vi "Create.vi"(6 "Shared Library":path=path "", 7 "Flags":i32, 8 "Error In":errorcluster) -> (0 "Error Out":errorcluster, 3 "LabSSH2":refnum<class "Context.lvclass">)   [LabVIEW 2017, in "LabSSH2.lvlib" / "Context.lvclass"]
uses:
  Context.lvclass
  Context.lvclass/Context.ctl
  LabSSH2.lvlib
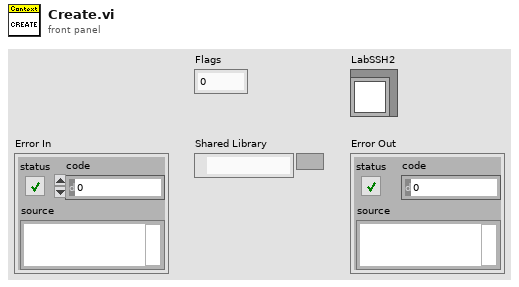
[diagram p1: front panel]
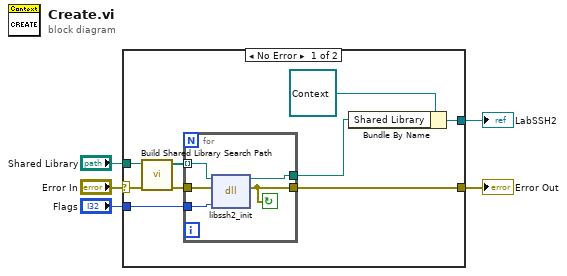
[diagram p0: block diagram]
diagram:
  n1 = case shown="No Error" "Error In" {
    selector: "Error In" -> [w14 w20]
    tunnel: "Shared Library" -> [w13 _]
    tunnel: [w7 w20] -> w3
    tunnel: [w8 _] -> w2
    tunnel: "Flags" -> [w6 _]
    frame No Error {
      n2 = call "Build Shared Library Search Path.vi"("Error In"=w14, "libssh2 Shared Library"=w13) -> ("Error Out"=w11:errorcluster, "Search Path"=w12:path[])  [unwired: 8 in]
      n3 = for {
        tunnel: w12 -> [w18] mode=indexing
        tunnel: w11 -> [w19]
        tunnel: [w17] -> w9
        tunnel: [w16] -> w7
        tunnel: w6 -> [w15]
        stop <- w16 continue-if-true
        n4 = dll-call lib="C:/Program Files/libssh2/bin/libssh2.dll" fn="libssh2_init"(path in=w18, error in=w19, "flags"=w15) -> (path out=w17:path, error out=w16:errorcluster)  [unwired: 3 in]
      }
      n5 = Bundle By Name(cluster=refnum<class "Context.lvclass"> refnum ("LabSSH2.lvlib:Context.lvclass"), "Shared Library"=w9) -> (w8:refnum<class "Context.lvclass">)
    }
    frame Error {
    }
  }
  "Error Out" <- w3
  "LabSSH2" <- w2
